vi "SetKeyValue.vi"(6 "value":string, 9 "key":string, 10 "key value pairs":T1[](array[typedef])) -> (2 "key value pairs out":T1[](array[typedef]))   [LabVIEW 2017, in "PropertyHelpers.lvlib"]
doc: "Writes the string value of a particular property or key in an array of key-value pairs. This VI is useful for defining properties that the device sends to NI InsightCM Server in the form of key-value pairs within NI InsightCM message bus messages."
uses:
  <vilib>/addons/InsightCM/Utilities/PropertyHelpers/PropertyHelpers.lvlib
  <vilib>/addons/InsightCM/MessageBus/Base/controls/KeyValuePair.ctl
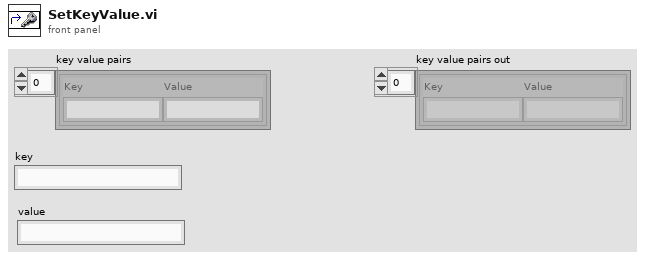
[diagram p1: front panel]
types:
  T1 = typedef "KeyValuePair.ctl" = cluster{"Key":string, "Value":string}
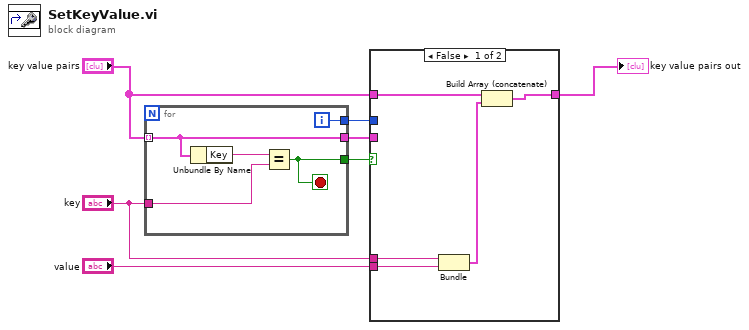
[diagram p0: block diagram]
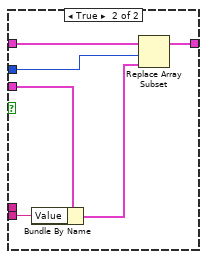
[diagram p2: hidden frame]
diagram:
  n1 = for {
    tunnel: "key value pairs" -> [w9] mode=indexing
    tunnel: "key" -> [w11]
    tunnel: [w10] -> w7
    tunnel: [w9] -> w6
    tunnel: [w8] -> w5
    i -> [w8]
    stop <- w10 stop-if-true
    n2 = Unbundle By Name(w9) -> ("Key"=w12:string)
    n3 = Equal?(x=w12, y=w11) -> (x = y?=w10:bool)
  }
  n4 = case shown="False" w7 {
    tunnel: w6 -> [_ w23]
    tunnel: "value" -> [w16 w22]
    tunnel: w5 -> [_ w21]
    tunnel: "key value pairs" -> [w17 w19]
    tunnel: [w14 w18] -> w4
    tunnel: "key" -> [w13 _]
    frame False {
      n5 = Bundle("key"=w13, "value"=w16) -> (w15:cluster{"key":string, "value":string})  [unwired: 1 in]
      n6 = Build Array (concatenate)(w17, w15) -> (w14:T1[])
    }
    frame True {
      n7 = Bundle By Name(cluster=w23, "Value"=w22) -> (w20:T1)
      n8 = Replace Array Subset(array=w19, new element=w20, index=w21) -> (w18:T1[])
    }
  }
  "key value pairs out" <- w4
